vi "JoystickSpeedControlTest.vi"() -> ()   [LabVIEW 2021, in "Test VIs.lvclass"]
uses:
  Test VIs/Test VIs.lvclass
  Drivers/Aerotech A3200/Parameters/SetAxisParameterDouble.vi
  Classes/Controller/Controller.lvclass
  Drivers/Aerotech A3200/Aerotech.lvlib
panel:
  out "error out":errorcluster
  in  "error in (no error)":errorcluster
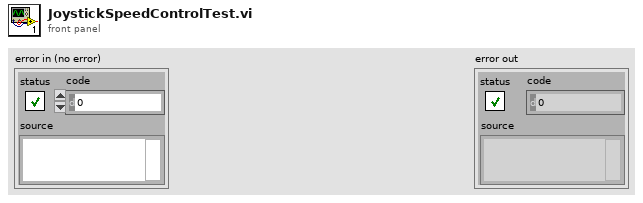
[diagram p1: front panel]
types:
  T1 = typedef "Controller.lvclass/Controllers.ctl" = cluster{"I-O.lvclass":refnum<class "I-O.lvclass">, "Gantry":refnum<k24>, "Dispenser":refnum<visa-resource-name>}
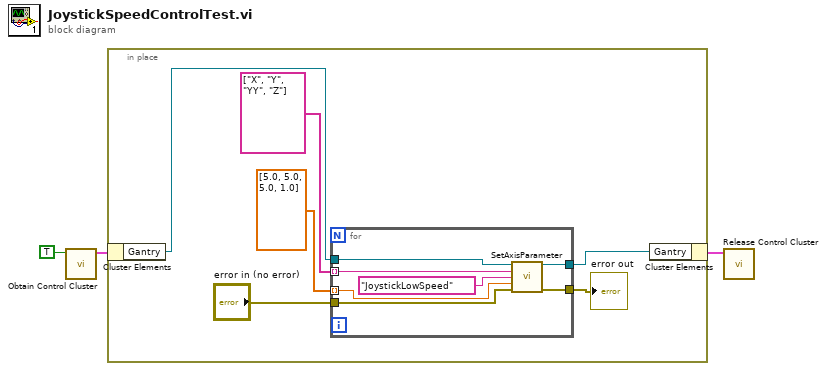
[diagram p0: block diagram]
diagram:
  n1 = call "Obtain Control Cluster.vi"("Motion"=TRUE) -> ("Control Out"=w2:T1)  [unwired: 9 in, 1 out]
  n2 = in-place {
    n3 = in-place-cluster #1(w2) -> ("Gantry"=w9:refnum<k24>)
    n4 = for {
      tunnel: w9 -> [w16]
      tunnel: "error in (no error)" -> [w14]
      tunnel: [w13] -> w7
      tunnel: [w12] -> w6
      tunnel: string[] ["X", "Y", "YY", "Z"] ("axisName") -> [w11] mode=indexing
      tunnel: dbl[] [5.0, 5.0, 5.0, 1.0] ("value") -> [w10] mode=indexing
      n5 = call-poly "SetAxisParameter.vi"("Controller In"=w16, "axisName"=w11, "Parameter Name"="JoystickLowSpeed", "value"=w10, "error in (no error)"=w14) -> ("Controller Out"=w13:refnum<k24>, "error out"=w12:errorcluster)  [unwired: 9 in]
    }
    "error out" <- w6
    n6 = in-place-cluster #1("Gantry"=w7) -> (w1:T1)
  }
  n7 = call "Release Control Cluster.vi"("output cluster"=w1) -> ()  [unwired: 11 in]
